vi "Comm Close.vi"(8 "error in (no error)":errorcluster {"code" format="%.0x"}, 11 "Device ID (0)":i32) -> (0 "error out":errorcluster {"code" format="%.0x"}, 2 "Return Code":i32, 3 "Device ID out":i32)   [LabVIEW 2020, in "KEYENCE LJ-X8000A.lvlib"]
uses:
  KEYENCE LJ-X8000A.lvlib
panel:
  # "(c) 2019 KEYENCE CORPORATION.  ALL RIGHTS RESERVED."
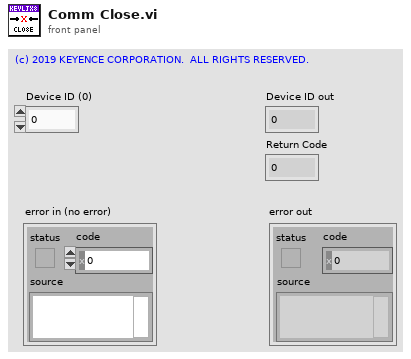
[diagram p1: front panel]
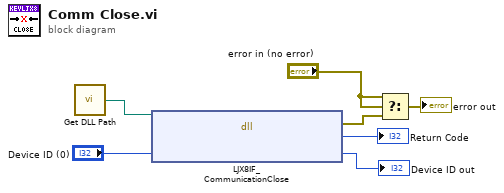
[diagram p0: block diagram]
diagram:
  n1 = call "Get DLL Path.vi"() -> ("DLL Path"=w1:path)  [unwired: 3 in]
  n2 = dll-call lib="C:/Program Files (x86)/National Instruments/LabVIEW 2018/instr.lib/KEYENCE LJ-X8000/LJX8_IF.*" fn="LJX8IF_CommunicationClose"(path in=w1, "lDeviceId"="Device ID (0)") -> (error out=w3:errorcluster, "lRetCode"=→"Return Code":i32, "lDeviceId"=→"Device ID out":i32)  [unwired: 2 in, 1 out]
  n3 = Select(t="error in (no error)", s="error in (no error)", f=w3) -> (s? t:f=→"error out":errorcluster)
